vi "GetMIMETypes.vi"(8 "error in (no error)":errorcluster, 11 "Config File":path) -> (0 "error out":errorcluster, 5 "MIME Types":variant)   [LabVIEW 2023]
uses:
  <vilib>/Utility/config.llb/Write Key (String).vi
  <vilib>/Utility/config.llb/Read Key (String).vi
  <vilib>/Utility/config.llb/NI_LVConfig.lvlib
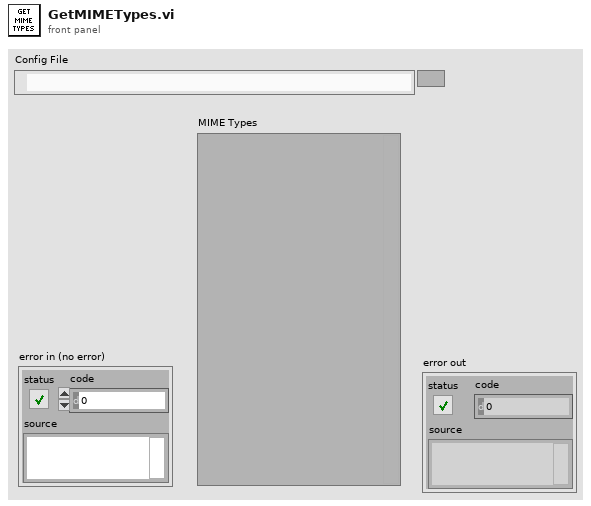
[diagram p1: front panel]
types:
  T1 = typedef "NI_LVConfig.lvlib/Config Data RefNum.ctl" = refnum<k1>
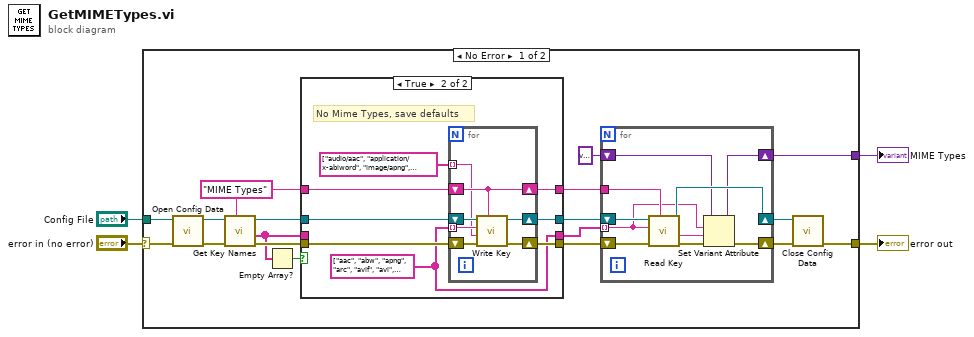
[diagram p0: block diagram]
diagram:
  n1 = case shown="No Error" "error in (no error)" {
    selector: "error in (no error)" -> [w22 w52]
    tunnel: "Config File" -> [w21 _]
    tunnel: [w16 w52] -> w2
    tunnel: [w14 _] -> w1
    frame No Error {
      w11 = "MIME Types" ("section")
      n2 = call <vilib>:"Open Config Data.vi"("error in (no error)"=w22, "configuration file path"=w21) -> ("error out"=w20:errorcluster, "refnum"=w19:T1)  [unwired: 7 in, 1 out]
      n3 = call <vilib>:"Get Key Names.vi"("section"=w11, "error in (no error)"=w20, "refnum"=w19) -> ("error out"=w12:errorcluster, "key names"=w7:string[], "refnum out"=w8:T1)  [unwired: 5 in, 1 out]
      n4 = Empty Array?(array=w7) -> (empty?=w13:bool)
      n5 = case shown="True" w13 {
        tunnel: w12 -> [w25 w34]
        tunnel: w11 -> [w23 w33]
        tunnel: [w26 w32] -> w10
        tunnel: [w25 w31] -> w9
        tunnel: w8 -> [w26 w30]
        tunnel: w7 -> [w24 _]
        tunnel: [w24 w27] -> w6
        tunnel: [w23 w29] -> w5
        frame False {
        }
        frame True {
          w27 = string[] ["aac", "abw", "apng", "arc", "avif", "avi", "azw", "bin", "bmp", "bz", "bz2", "cda", "csh", "css", "csv", "doc", "docx", "eot", "epub", "gz", "gif", "htm", "html", "ico", "ics", "jar", "jpeg, .jpg", "js", "json", "jsonld", "md", "mid", "midi", "mjs", "mp3", "mp4", "mpeg", "mpkg", "odp", "ods", "odt", "oga", "ogv", "ogx", "opus", "otf", "png", "pdf", "php", "ppt", "pptx", "rar", "rtf", "sh", "svg", "tar", "tif, .tiff", "ts", "ttf", "txt", "vsd", "wav", "weba", "webm", "webmanifest", "webp", "woff", "woff2", "xhtml", "xls", "xlsx", "xml", "xul", "zip", "3gp", "3g2", "7z"] ("Ext")
          # "No Mime Types, save defaults"
          n6 = for {
            shift-right: [w39] -> w31
            shift-left: w34 -> [w40]
            shift-right: [w38] -> w32
            shift-left: w30 -> [w41]
            shift-right: [w37] -> w29
            shift-left: w33 -> [w37]
            tunnel: w27 -> [w36] mode=indexing
            tunnel: string[] ["audio/aac", "application/x-abiword", "image/apng", "application/x-freearc", "image/avif", "video/x-msvideo", "application/vnd.amazon.ebook", "application/octet-stream", "image/bmp", "application/x-bzip", "application/x-bzip2", "application/x-cdf", "application/x-csh", "text/css", "text/csv", "application/msword", "application/vnd.openxmlformats-officedocument.wordprocessingml.document", "application/vnd.ms-fontobject", "application/epub+zip", "application/gzip", "image/gif", "text/html", "text/html", "image/vnd.microsoft.icon", "text/calendar", "application/java-archive", "image/jpeg", "text/javascript", "application/json", "application/ld+json", "text/markdown", "audio/midi", "audio/x-midi", "text/javascript", "audio/mpeg", "video/mp4", "video/mpeg", "application/vnd.apple.installer+xml", "application/vnd.oasis.opendocument.presentation", "application/vnd.oasis.opendocument.spreadsheet", "application/vnd.oasis.opendocument.text", "audio/ogg", "video/ogg", "application/ogg", "audio/ogg", "font/otf", "image/png", "application/pdf", "application/x-httpd-php", "application/vnd.ms-powerpoint", "application/vnd.openxmlformats-officedocument.presentationml.presentation", "application/vnd.rar", "application/rtf", "application/x-sh", "image/svg+xml", "application/x-tar", "image/tiff", "video/mp2t", "font/ttf", "text/plain", "application/vnd.visio", "audio/wav", "audio/webm", "video/webm", "application/manifest+json", "image/webp", "font/woff", "font/woff2", "application/xhtml+xml", "application/vnd.ms-excel", "application/vnd.openxmlformats-officedocument.spreadsheetml.sheet", "application/xml", "application/vnd.mozilla.xul+xml", "application/zip", "video/3gpp", "video/3gpp2", "application/x-7z-compressed"] ("mimetype") -> [w35] mode=indexing
            n7 = call-poly <vilib>:"Write Key.vi"("section"=w37, "error in (no error)"=w40, "value"=w35, "key"=w36, "refnum"=w41) -> ("error out"=w39:errorcluster, "refnum out"=w38:T1)  [unwired: 4 in, 1 out]
          }
        }
      }
      n8 = for {
        shift-right: [w46] -> w17
        shift-left: w9 -> [w50]
        shift-right: [w48] -> w18
        shift-left: w10 -> [w51]
        tunnel: w6 -> [w43] mode=indexing
        tunnel: w5 -> [w49]
        shift-right: [w44] -> w14
        shift-left: variant -> [w45]
        n9 = call-poly <vilib>:"Read Key.vi"("section"=w49, "error in (no error)"=w50, "key"=w43, "refnum"=w51) -> ("error out"=w47:errorcluster, "value"=w42:string, "refnum out"=w48:T1)  [unwired: 4 in, 1 out]
        n10 = Set Variant Attribute(Variant=w45, name=w43, value=w42, error in=w47) -> (Variant out=w44:variant, error out=w46:errorcluster)  [unwired: 1 out]
      }
      n11 = call <vilib>:"Close Config Data.vi"("error in (no error)"=w17, "refnum"=w18) -> ("error out"=w16:errorcluster)  [unwired: 8 in, 1 out]
    }
    frame Error {
    }
  }
  "error out" <- w2
  "MIME Types" <- w1
